vi "Measurement.WavelengthSweeping.UI.GetDependencies.vi"(8 "error in (no error)":errorcluster, 11 "Measurement.PhotocurrentMapping.UI in":refnum<class "Measurement.PhotocurrentMapping.UI.lvclass">) -> (0 "error out":errorcluster, 2 "Dependencies":T1, 3 "Measurement.PhotocurrentMapping.UI out":refnum<class "Measurement.PhotocurrentMapping.UI.lvclass">)   [LabVIEW 2017, in "Measurement.PhotocurrentMapping.UI.lvclass"]
uses:
  Measurement.PhotocurrentMapping.UI.lvclass
  Typedefs/Dependencies--Cluster.ctl
  Measurement.PhotocurrentMapping/Measurement.PhotocurrentMapping.lvclass
  Measurement.PhotocurrentMapping.UI.lvclass/Measurement.PhotocurrentMapping.UI.ctl
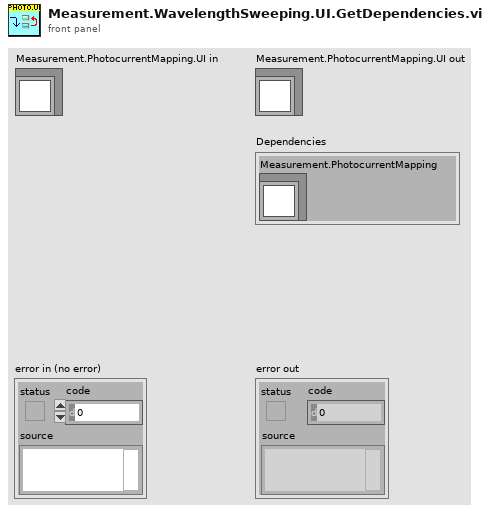
[diagram p1: front panel]
types:
  T1 = typedef "Measurement.PhotocurrentMapping.UI.lvclass/Dependencies--Cluster.ctl" = cluster{"Measurement.PhotocurrentMapping":refnum<class "Measurement.PhotocurrentMapping.lvclass">}
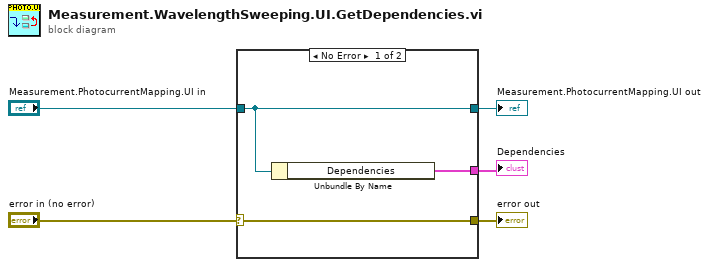
[diagram p0: block diagram]
diagram:
  n1 = case shown="No Error" "error in (no error)" {
    selector: "error in (no error)" -> [w8 w10]
    tunnel: [w8 w10] -> w4
    tunnel: [w7 w9] -> w2
    tunnel: "Measurement.PhotocurrentMapping.UI in" -> [w7 w9]
    tunnel: [w6 _] -> w1
    frame No Error {
      n2 = Unbundle By Name(w7) -> ("Dependencies"=w6:T1)
    }
    frame Error {
    }
  }
  "error out" <- w4
  "Measurement.PhotocurrentMapping.UI out" <- w2
  "Dependencies" <- w1
